vi "cluster-head-to-array.vi"(4 "cluster ref":refnum<vi>) -> (7 "Labels":string[](array[string]))   [LabVIEW 2011]
panel:
  out "Label.Text":string
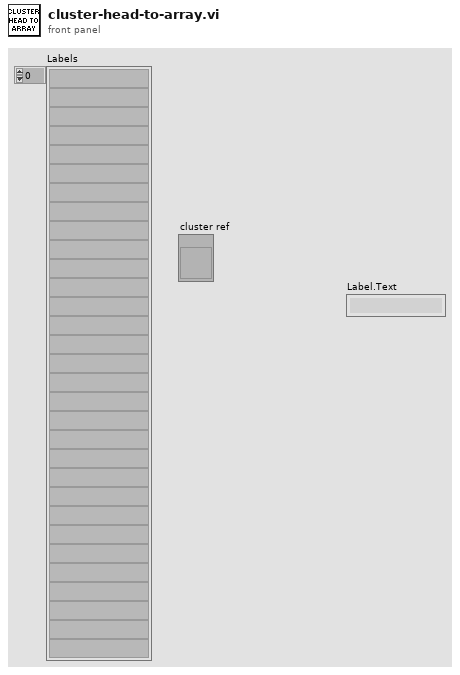
[diagram p1: front panel]
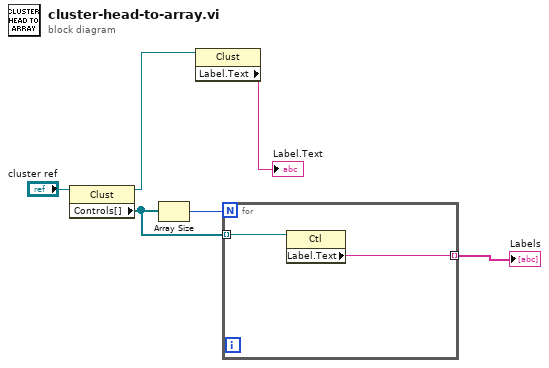
[diagram p0: block diagram]
diagram:
  n1 = property class="Clust"(reference="cluster ref") -> (reference out=w6:refnum<vi>, "Controls[]"=w4:refnum<vi>[])  [unwired: 1 in, 1 out]
  n2 = Array Size(array=w4) -> (size(s)=w3:i32)
  n3 = property class="Clust"(reference=w6) -> ("Label.Text"=→"Label.Text":string)  [unwired: 1 in, 2 out]
  n4 = for {
    N: w3 -> [_]
    tunnel: w4 -> [w8] mode=indexing
    tunnel: [w7] -> w2 mode=indexing
    n5 = property class="Ctl"(reference=w8) -> ("Label.Text"=w7:string)  [unwired: 1 in, 2 out]
  }
  "Labels" <- w2
